vi "RefreshXYGraph.vi"(8 "error in (no error)":errorcluster caption="entrée d'erreur (pas d'erreur)", 9 "Graph Index":i32, 11 "Interface en entrée":refnum<class "Interface.lvclass"> caption="DNL_LabVIEW Object in") -> (0 "error out":errorcluster caption="sortie d'erreur", 1 "CurvesInd":i32[](array[numeric]), 3 "Interface en sortie":refnum<class "Interface.lvclass"> caption="DNL_LabVIEW Object out")   [LabVIEW 2019, in "Interface.lvclass"]
uses:
  Interface.lvclass
  Interface.lvclass/Interface.ctl
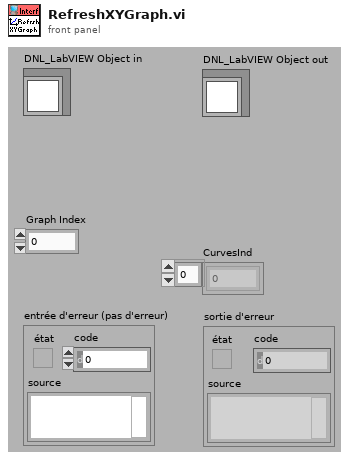
[diagram p1: front panel]
types:
  T1 = cluster{"Message":string, "Data":variant, i32, cluster{dbl[], dbl[]}[]}
  T2 = typedef "Interface.lvclass/CurveSetup.ctl" = cluster{"CurveName":string, "YParam":string, "XParam":string, "ZParam ":string, "GroupName":string, "LinWdth":u8, "PntCol":u32, "LinCol":u32, "LablFor":u8, "XScale":u32, "YScale":u32, "Interpol":u8, "DisplayName":string, "FillType":i16, "LineStyle":u8, "PntStyle":u8, "BarTyp":u8, "GraphIndex":i32, "Visible":bool, "XScaleName":string, "YScaleName":string, "XYGraph_Ref":refnum<vi>, "Data Only":bool, "DataQ Ref":refnum<queue>, "XParQ Ref":refnum<queue>, "XParamInd":i32, "ScanInd":i32, "File Path":path}
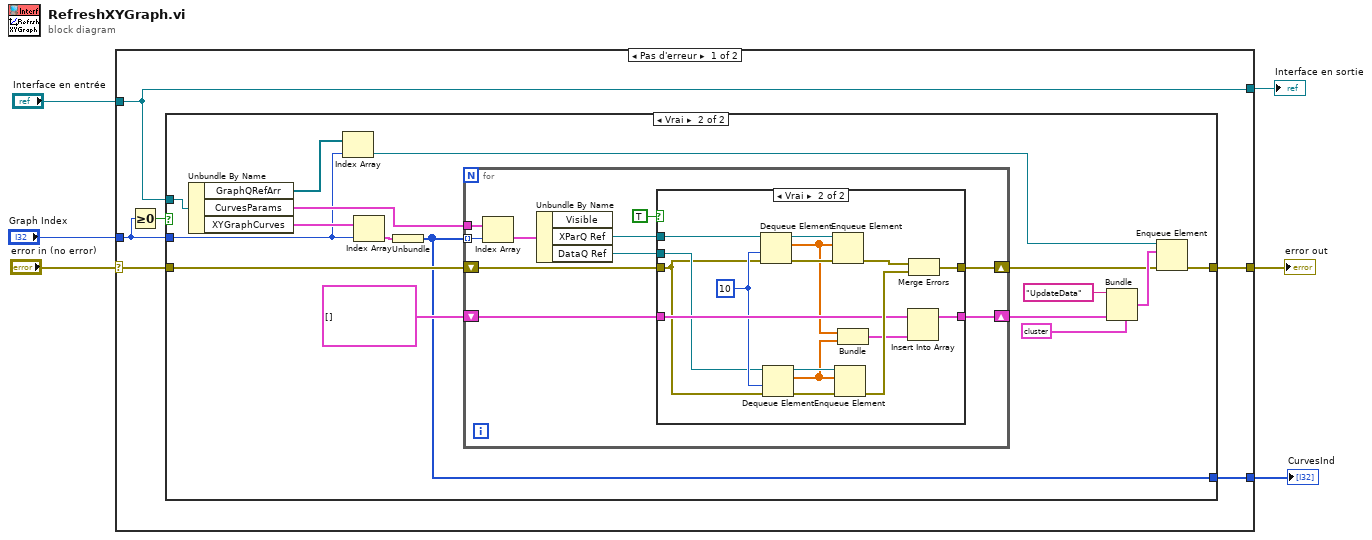
[diagram p0: block diagram]
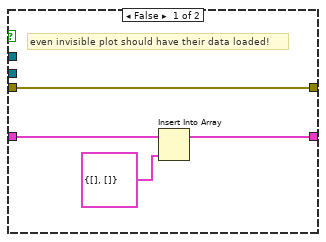
[diagram p3: hidden frame]
diagram:
  n1 = case shown="Pas d'erreur" "error in (no error)" {
    selector: "error in (no error)" -> [w11 w61]
    tunnel: [w10 w61] -> w5
    tunnel: [w12 w60] -> w3
    tunnel: "Interface en entrée" -> [w12 w60]
    tunnel: [w9 _] -> w2
    tunnel: "Graph Index" -> [w8 _]
    frame No Error {
      n2 = Greater Or Equal To 0?(x=w8) -> (x >= 0?=w7:bool)
      n3 = case shown="Vrai" w7 {
        tunnel: w12 -> [_ w29]
        tunnel: w11 -> [w13 w28]
        tunnel: [w13 w22] -> w10
        tunnel: [_ w25] -> w9
        tunnel: w8 -> [_ w20]
        frame False {
        }
        frame True {
          n4 = Unbundle By Name(w29) -> ("GraphQRefArr"=w14:refnum<queue>[], "CurvesParams"=w23:T2[], "XYGraphCurves"=w24:cluster{"Tableau":i32[]}[])
          n5 = Index Array(array=w14, index=w20) -> (element=w21:refnum<queue>)
          n6 = Index Array(array=w24, index=w20) -> (element=w27:cluster{"Tableau":i32[]})
          n7 = Unbundle(w27) -> ("Tableau"=w25:i32[])
          n8 = for {
            tunnel: w25 -> [w38] mode=indexing
            shift-right: [w31] -> w17
            shift-left: w28 -> [w32]
            tunnel: w23 -> [w39]
            shift-right: [w34] -> w16
            shift-left: cluster{dbl[], dbl[]}[] [] -> [w35]
            n9 = Index Array(array=w39, index=w38) -> (element=w37:T2)
            n10 = Unbundle By Name(w37) -> ("XParQ Ref"=w33:refnum<queue>, "DataQ Ref"=w36:refnum<queue>)  [unwired: 1 out]
            n11 = case shown="Vrai" TRUE {
              tunnel: w33 -> [_ w50]
              tunnel: w36 -> [_ w49]
              tunnel: w32 -> [w43 w48]
              tunnel: [w42 w54] -> w34
              tunnel: [w43 w51] -> w31
              tunnel: w35 -> [w41 w53]
              frame False {
                # "even invisible plot should have their data loaded!"
                n12 = Insert Into Array(array=w41, new element=cluster{dbl[], dbl[]} {[], []} ("nouvel élément/sous-tableau")) -> (w42:cluster{dbl[], dbl[]}[])  [unwired: 1 in]
              }
              frame True {
                w52 = 10 ("timeout en ms (-1)")
                n13 = Dequeue Element(queue=w50, timeout in ms (-1)=w52, error in (no error)=w48) -> (queue out=w59:refnum<queue>, element=w45:dbl[], error out=w47:errorcluster)  [unwired: 1 out]
                n14 = Dequeue Element(queue=w49, timeout in ms (-1)=w52, error in (no error)=w48) -> (queue out=w56:refnum<queue>, element=w44:dbl[], error out=w57:errorcluster)  [unwired: 1 out]
                n15 = Enqueue Element(queue=w59, element=w45, error in (no error)=w47) -> (error out=w58:errorcluster)  [unwired: 1 in, 2 out]
                n16 = Enqueue Element(queue=w56, element=w44, error in (no error)=w57) -> (error out=w55:errorcluster)  [unwired: 1 in, 2 out]
                n17 = Bundle(w45, w44) -> (w46:cluster{dbl[], dbl[]})  [unwired: 1 in]
                n18 = Insert Into Array(array=w53, new element=w46) -> (w54:cluster{dbl[], dbl[]}[])  [unwired: 1 in]
                n19 = Merge Errors(w58, w55) -> (w51:errorcluster)
              }
            }
          }
          n20 = Bundle(cluster=T1 {"Message"="", "Data"=variant, 0, []} ("élément"), "Message"="UpdateData", w16) -> (w18:T1)  [unwired: 2 in]
          n21 = Enqueue Element(queue=w21, element=w18, error in (no error)=w17) -> (error out=w22:errorcluster)  [unwired: 1 in, 2 out]
        }
      }
    }
    frame Error {
    }
  }
  "error out" <- w5
  "Interface en sortie" <- w3
  "CurvesInd" <- w2
